vi "vkri801 Assignment_1_XY_Platform.vi"() -> ()   [LabVIEW 2015]
uses:
  <vilib>/DAQmx/create/channels.llb/DAQmx Create Channel (AO-Voltage-Basic).vi
  <vilib>/Utility/error.llb/DialogType.ctl
  <vilib>/DAQmx/create/channels.llb/DAQmx Create Channel (DI-Digital Input).vi
  <vilib>/DAQmx/write.llb/DAQmx Write (Analog DBL 1Chan 1Samp).vi
  <vilib>/DAQmx/read.llb/DAQmx Read (Digital Bool 1Line 1Point).vi
panel:
  in  "Tab Control 2":enum32{"Logistics button"}(tab)
  in  "Motor On/Off":bool
  in  "STOP":bool
  in  "Centre Switch":bool
  in  "Tab Control":enum32{"Pulse Width Graphs"}(tab)
  out "Pulses Left Encoder":dynamicdata(graph) caption="Square"
  out "Pulses Right Encoder":dynamicdata(graph) caption="Square"
  in  "Pulse Width Reset":bool
  in  "Speed Gauges":T1(tab)
  out "Speed Right Motor mm/s":dbl(knob) scale=-50.0..50.0 scale format="%#_6p"
  out "Speed Left Motor mm/s":dbl(knob) scale=-50.0..50.0 scale format="%#_6p"
  out "Y Dimension Speed mm/s 2":dbl(knob) scale=-50.0..50.0 scale format="%#_6p"
  out "X Dimension Speed mm/s 2":dbl(knob) scale=-50.0..50.0 scale format="%#_6p"
  out "LEFT RPM":dbl(knob) scale=-50.0..50.0 scale format="%#_6p"
  out "RIGHT RPM":dbl(knob) scale=-50.0..50.0 scale format="%#_6p"
  in  "Cradle Position":enum32{"Cradle Position"}(tab)
  out "XY Graph 2":cluster{dbl[], dbl[]}(graph)
  in  "Clear Graph":bool
  in  "Chart History":i32=500 caption="Maximum Number of Data Points (Chart History)"
  in  "Read outs":T2(tab)
  out "Left Motor Distance  (mm)":dbl
  out "Right Motor Distance  (mm)":dbl
  out "Right Motor Encoder":dbl
  out "Left Motor Encoder":dbl
  out "Left Motor Frequency":dbl
  out "Right Motor Frequency":dbl
  out "Y":dbl
  out "X":dbl
  out "Y Error":dbl
  out "X Error":dbl
  out "Cursor Y":dbl format="%.2f"
  out "Cursor X":dbl format="%.2f"
  out "X Circle":dbl
  out "Y Circle":dbl
  out "Right Motor Voltage":dbl
  out "Left Motor Voltage":dbl
  in  "Indicator LED":enum32{"Limit Switches"}(tab)
  out "Left":bool
  out "Right":bool
  out "Top":bool
  out "Bottom":bool
  in  "Controls Tab":T3(tab)
  in  "Top Button":bool
  in  "Right Button":bool
  in  "Left Button":bool
  in  "Down Button":bool
  in  "Speed Control":dbl(knob) scale=0.0..10.0
  in  "Left Motor Speed":dbl(knob) scale=-10.0..10.0
  in  "Right Motor Speed":dbl(knob) scale=-10.0..10.0
  in  "Max Voltage":dbl(knob) scale=0.0..10.0
  in  "XY Cursor Graph":cluster{dbl, dbl}[](graph)
  in  "Graph/Coordinate Execute":bool
  in  "K Gain Graph":dbl
  in  "Max Voltage Rectangle":dbl
  in  "Length":dbl
  in  "Width":dbl
  out "Top Left X":dbl
  out "Top Left Y":dbl
  in  "Draw Rectangle":bool
  in  "Y Gain Rectangle":dbl
  in  "X Gain Rectangle":dbl
  in  "Gain Rec":dbl
  in  "Rec Drift Fix":dbl
  in  "Draw Circle":bool
  in  "Reset Circle":bool
  in  "Radius":dbl=-15.0 caption="Amplitude"
  in  "Speed":dbl=0.01 caption="Frequency"
  in  "K Gain Circle":dbl
  in  "X Origin":dbl caption="Offset"
  in  "Y Origin":dbl caption="Offset"
  in  "Channel Selection and Limit Values":T4(tab)
  in  "Right Motor Channel (ao0)":tag="Dev4/ao0"
  in  "Bottom LED":tag="Dev4/ao0"
  in  "Right LED":tag="Dev4/ao0"
  in  "Left LED":tag="Dev4/ao0"
  in  "Left Motor Channel (ao1)":tag="Dev4/ao0"
  in  "Top LED":tag="Dev4/ao0"
  in  "Minimum Voltage":dbl=-6.0
  in  "Maximum Voltage":dbl=6.0
  in  "Rectangle Stop":bool
  in  "Left OK":bool
  in  "Up OK":bool
  in  "Right OK":bool
  in  "Centre Stop":bool
  in  "Numeric Right":dbl
  out "Pulses before refresh\nRight":dbl
  in  "Numeric Left":dbl
  out "Pulses before refresh\nLeft":dbl
  # "Vincent and Mohammad - XY Platform Software"
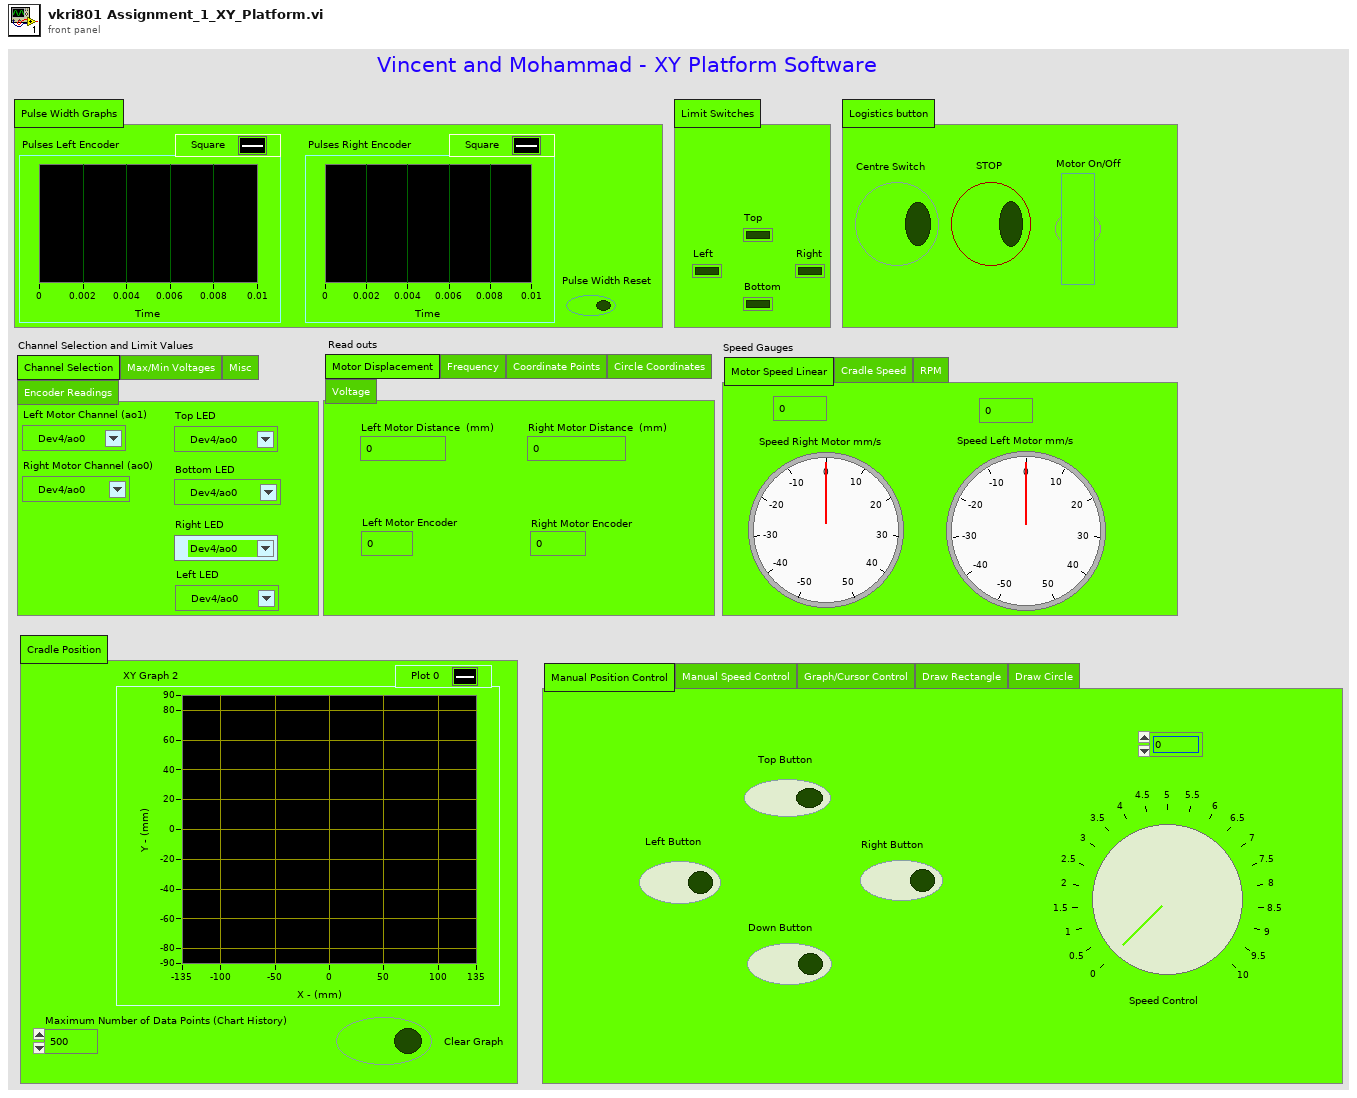
[diagram p1: front panel]
types:
  T1 = enum32{"Motor Speed Linear", "Cradle Speed", "RPM"}
  T2 = enum32{"Motor Displacement", "Frequency", "Coordinate Points", "Circle Coordinates", "Voltage"}
  T3 = enum32{"Manual Position Control", "Manual Speed Control", "Graph/Cursor Control", "Draw Rectangle", "Draw Circle"}
  T4 = enum32{"Channel Selection", "Max/Min Voltages", "Misc", "Encoder Readings"}
  T5 = typedef "DialogType.ctl" = u16
  T6 = typedef "LVPointDoubleTypeDef.ctl" = cluster{"Cursor X":dbl, "Cursor Y":dbl}
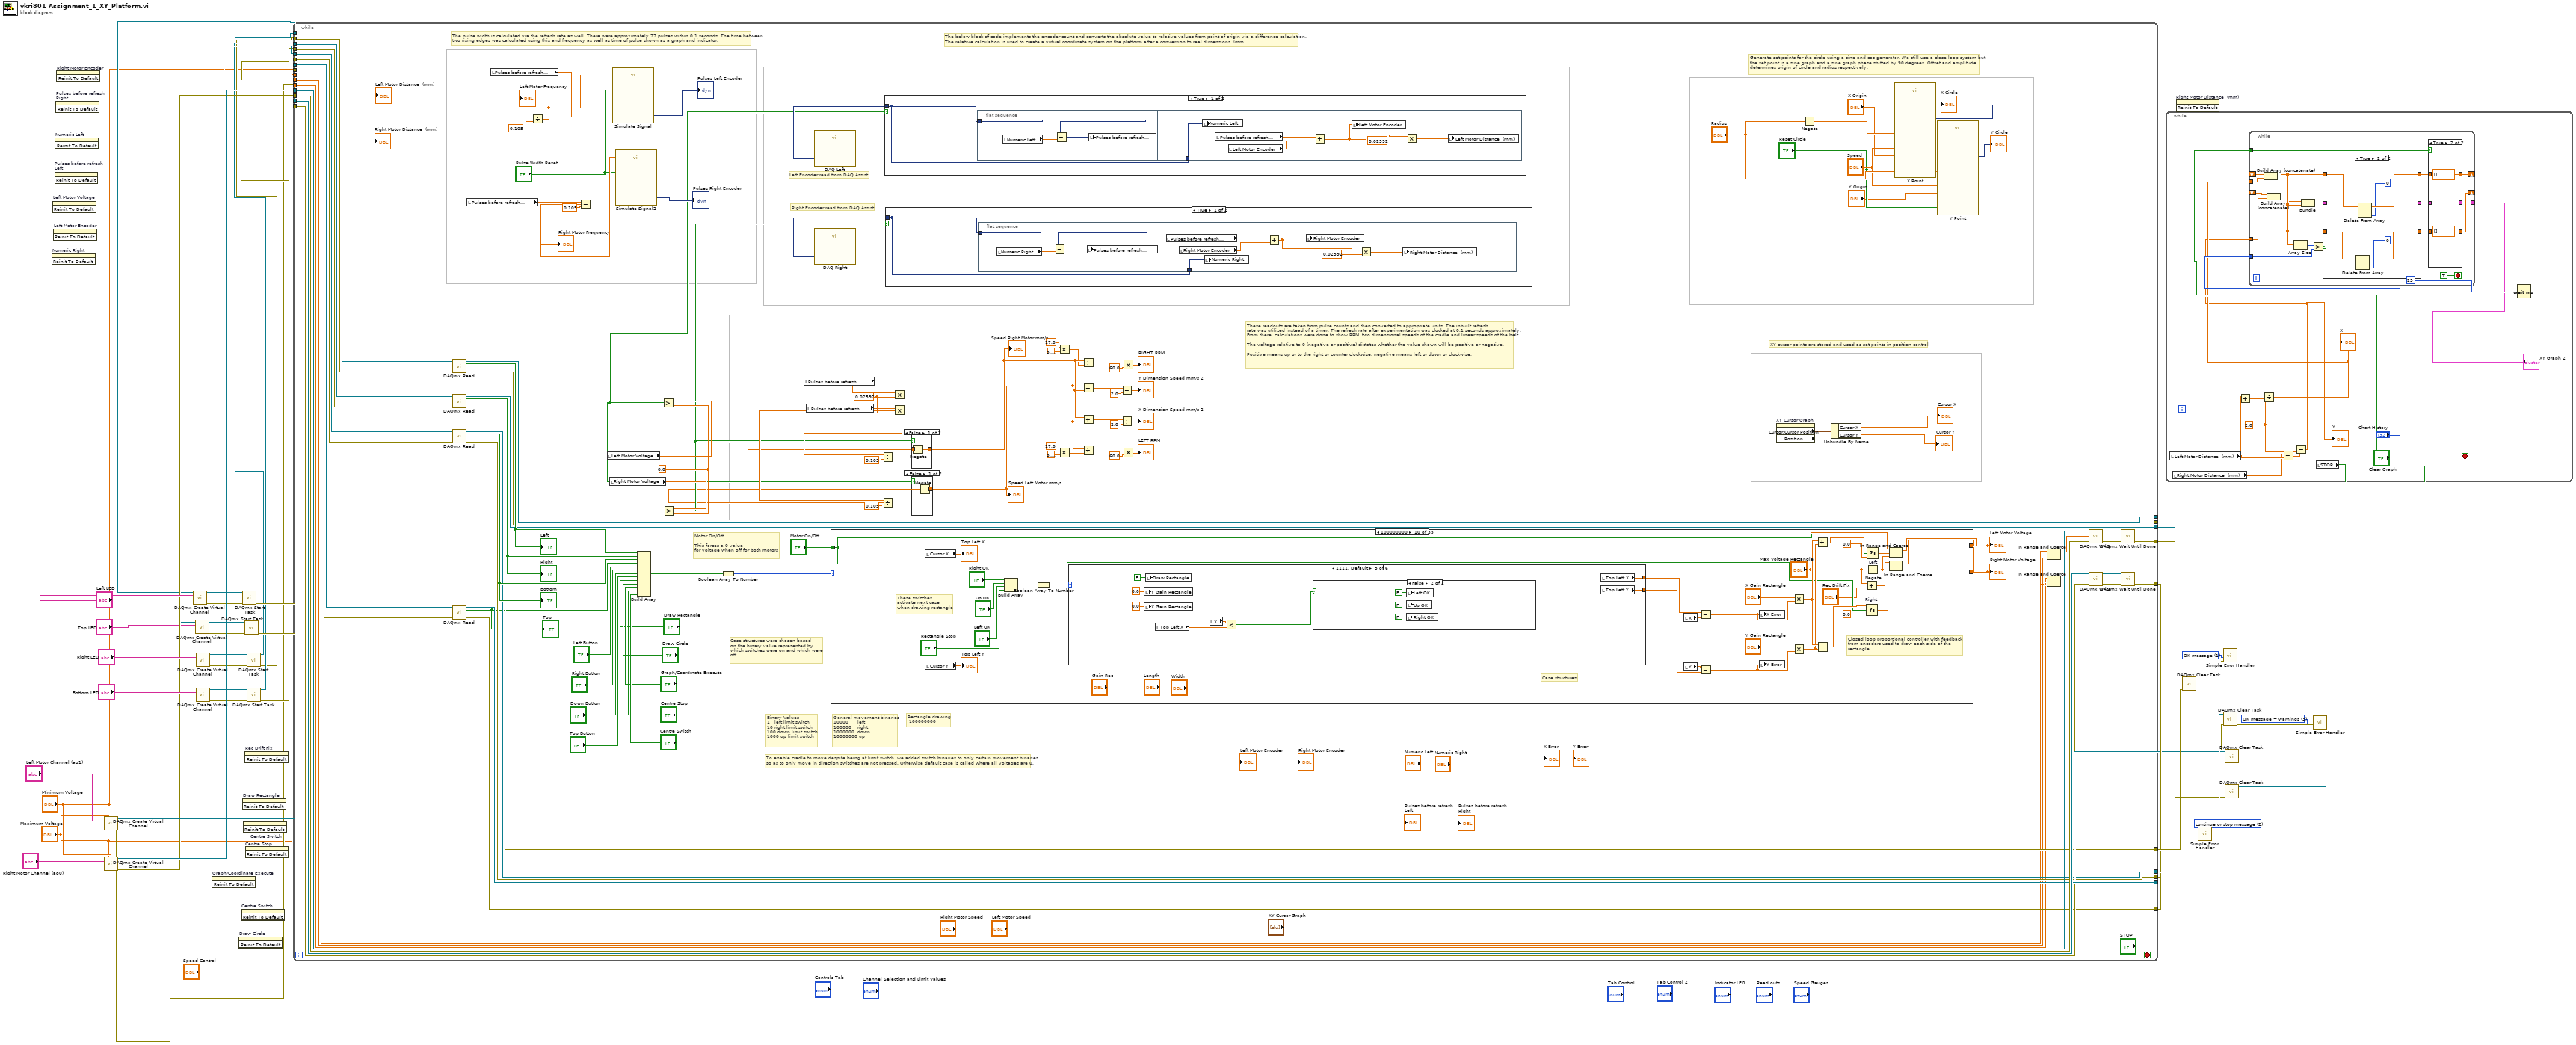
[diagram p0: block diagram]
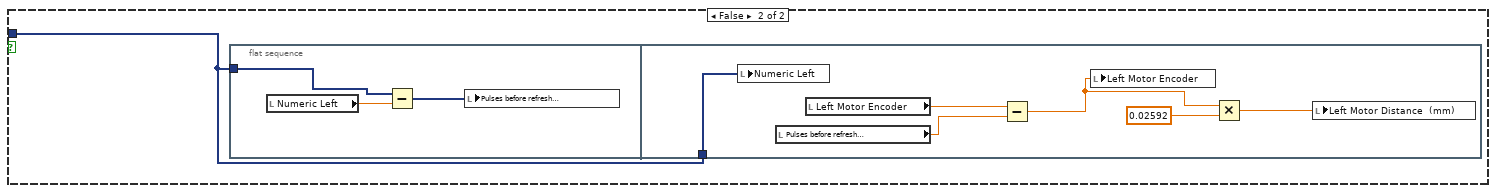
[diagram p6: hidden frame]
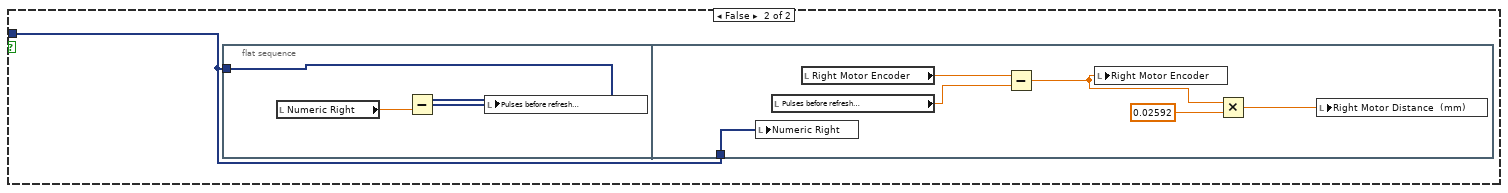
[diagram p7: hidden frame]
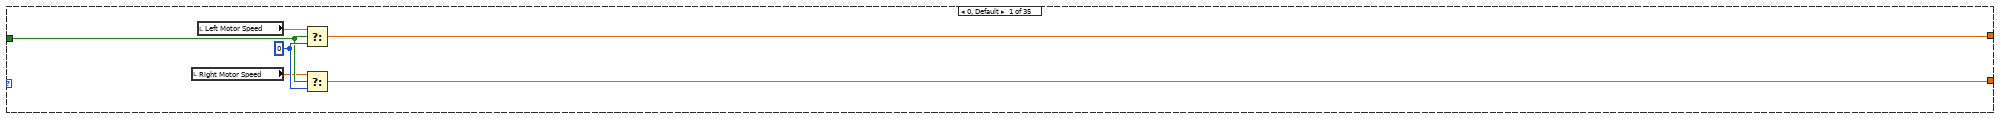
[diagram p8: hidden frame]
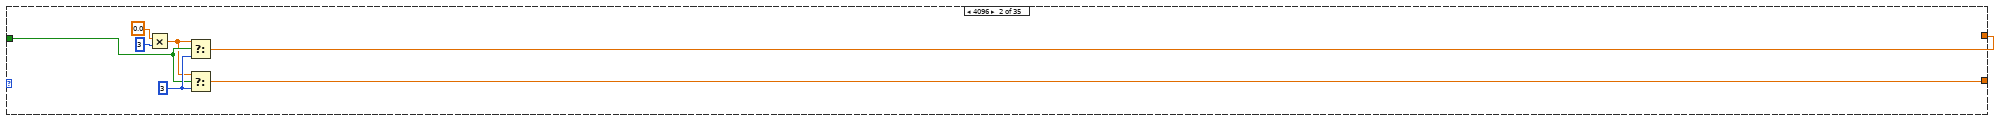
[diagram p9: hidden frame]
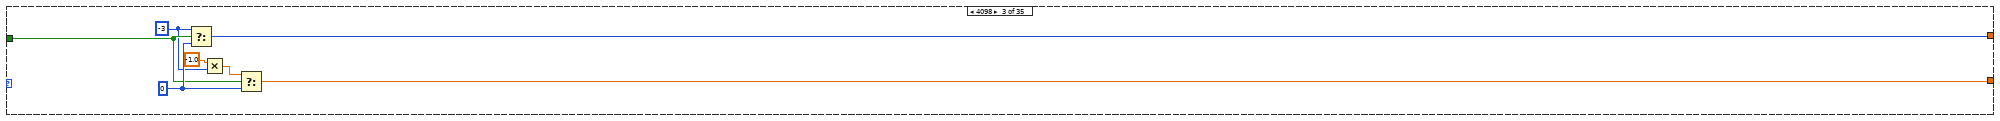
[diagram p10: hidden frame]
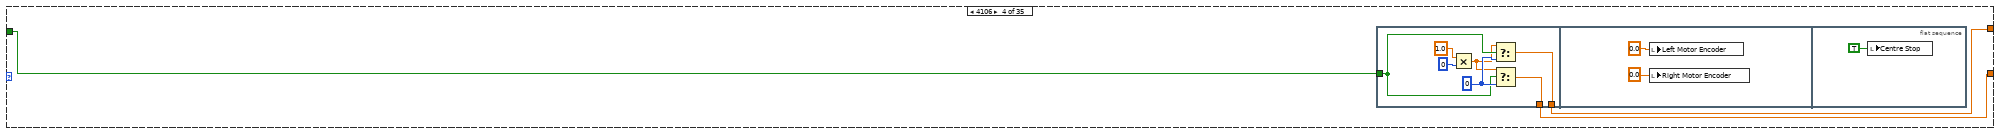
[diagram p11: hidden frame]
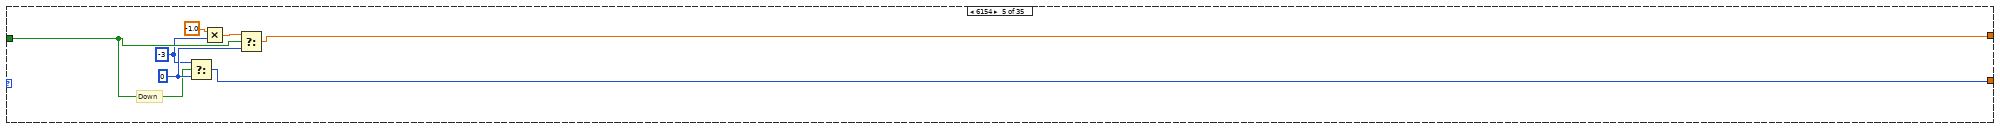
[diagram p12: hidden frame]
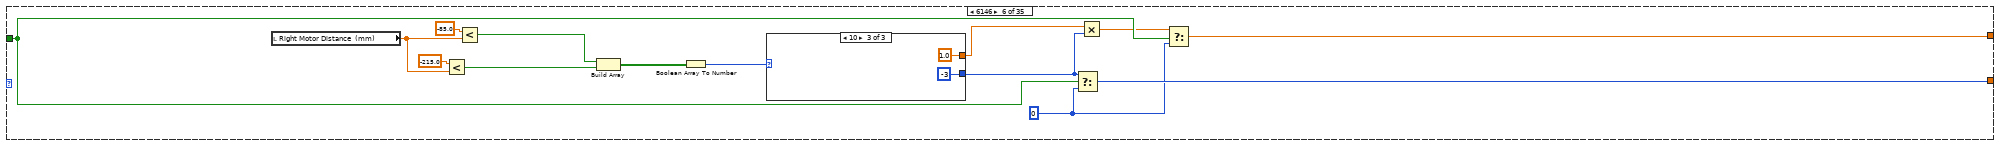
[diagram p13: hidden frame]
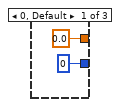
[diagram p14: hidden frame]
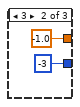
[diagram p15: hidden frame]
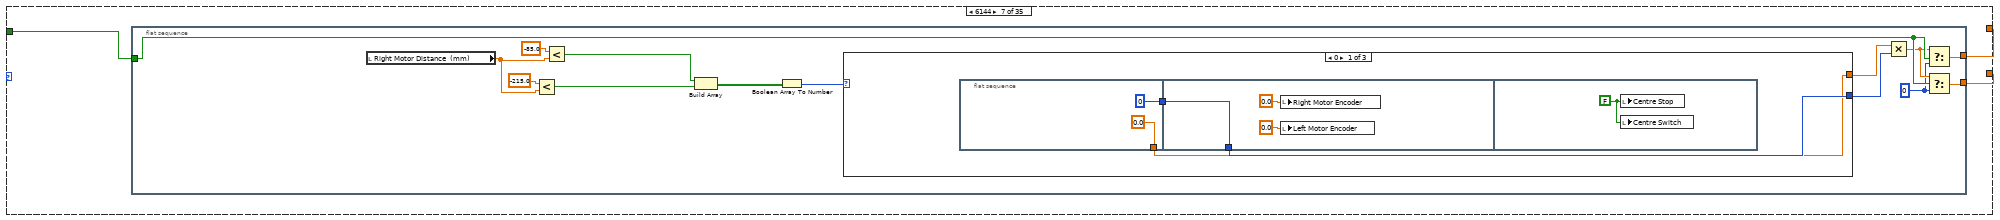
[diagram p16: hidden frame]
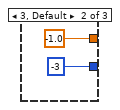
[diagram p17: hidden frame]
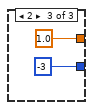
[diagram p18: hidden frame]
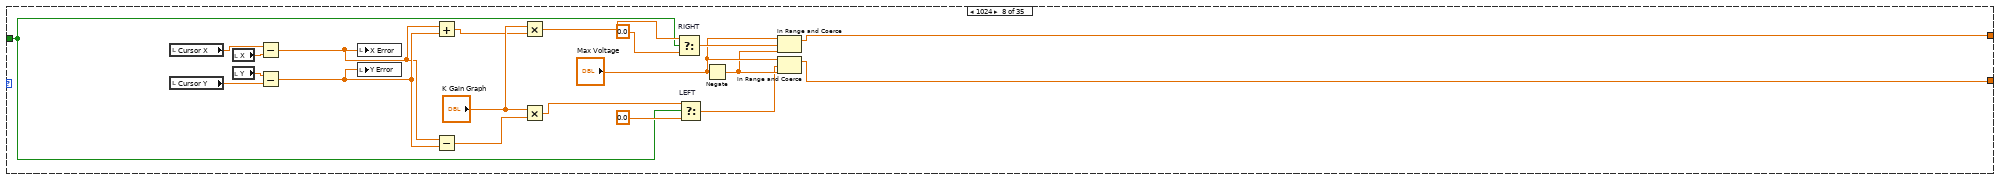
[diagram p19: hidden frame]
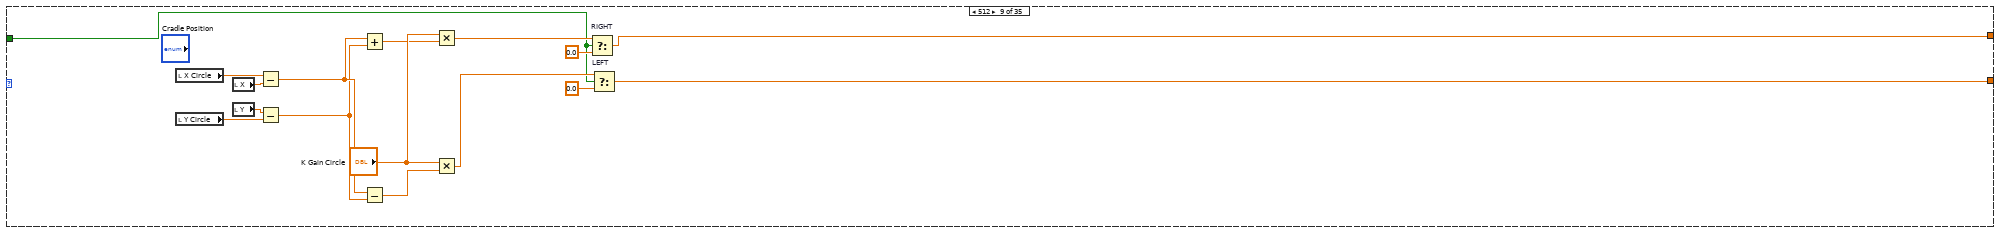
[diagram p20: hidden frame]
diagram:
  w24 = T5 3 items=["no dialog", "OK message", "continue or stop message", "OK message + warnings", "continue/stop + warnings"] ("type of dialog (OK msg:1)")
  w38 = T5 1 items=["no dialog", "OK message", "continue or stop message", "OK message + warnings", "continue/stop + warnings"] ("type of dialog (OK msg:1)")
  w42 = T5 2 items=["no dialog", "OK message", "continue or stop message", "OK message + warnings", "continue/stop + warnings"] ("type of dialog (OK msg:1)")
  n1 = invoke on="Numeric Right" class="DigNum (strict)" method="Reinit To Default"() -> ()  [unwired: 3 in, 3 out]
  n2 = invoke on="Left Motor Voltage" class="DigNum (strict)" method="Reinit To Default"() -> ()  [unwired: 3 in, 3 out]
  n3 = invoke on="Left Motor Encoder" class="DigNum (strict)" method="Reinit To Default"() -> ()  [unwired: 3 in, 3 out]
  n4 = invoke on="Pulses before refresh\nLeft" class="DigNum (strict)" method="Reinit To Default"() -> ()  [unwired: 3 in, 3 out]
  n5 = invoke on="Numeric Left" class="DigNum (strict)" method="Reinit To Default"() -> ()  [unwired: 3 in, 3 out]
  n6 = invoke on="Pulses before refresh\nRight" class="DigNum (strict)" method="Reinit To Default"() -> ()  [unwired: 3 in, 3 out]
  n7 = invoke on="Right Motor Encoder" class="DigNum (strict)" method="Reinit To Default"() -> ()  [unwired: 3 in, 3 out]
  n8 = call-poly <vilib>:"DAQmx Create Virtual Channel.vi"("maximum value"="Maximum Voltage", "minimum value"="Minimum Voltage", "physical channels"="Left Motor Channel (ao1)") -> ("task out"=w37:refnum<k21>, "error out"=w14:errorcluster)  [unwired: 11 in]
  n9 = call-poly <vilib>:"DAQmx Create Virtual Channel.vi"("maximum value"="Maximum Voltage", "minimum value"="Minimum Voltage", "physical channels"="Right Motor Channel (ao0)") -> ("task out"=w40:refnum<k21>, "error out"=w23:errorcluster)  [unwired: 11 in]
  n10 = call-poly <vilib>:"DAQmx Create Virtual Channel.vi"("lines"="Left LED") -> ("task out"=w26:refnum<k21>, "error out"=w27:errorcluster)  [unwired: 13 in]
  n11 = call-poly <vilib>:"DAQmx Create Virtual Channel.vi"("lines"="Top LED") -> ("task out"=w35:refnum<k21>, "error out"=w36:errorcluster)  [unwired: 13 in]
  n12 = call-poly <vilib>:"DAQmx Create Virtual Channel.vi"("lines"="Right LED") -> ("task out"=w29:refnum<k21>, "error out"=w30:errorcluster)  [unwired: 13 in]
  n13 = call-poly <vilib>:"DAQmx Create Virtual Channel.vi"("lines"="Bottom LED") -> ("task out"=w32:refnum<k21>, "error out"=w33:errorcluster)  [unwired: 13 in]
  n14 = invoke on="Graph/Coordinate Execute" class="Bool (strict)" method="Reinit To Default"() -> ()  [unwired: 3 in, 3 out]
  n15 = invoke on="Draw Circle" class="Bool (strict)" method="Reinit To Default"() -> ()  [unwired: 3 in, 3 out]
  n16 = invoke on="Centre Switch" class="Bool (strict)" method="Reinit To Default"() -> ()  [unwired: 3 in, 3 out]
  n17 = call <vilib>:"DAQmx Start Task.vi"("task/channels in"=w26, "error in"=w27) -> ("task out"=w21:refnum<k21>, "error out"=w22:errorcluster)  [unwired: 12 in]
  n18 = invoke on="Draw Rectangle" class="Bool (strict)" method="Reinit To Default"() -> ()  [unwired: 3 in, 3 out]
  n19 = invoke on="Centre Switch" class="Bool (strict)" method="Reinit To Default"() -> ()  [unwired: 3 in, 3 out]
  n20 = call <vilib>:"DAQmx Start Task.vi"("task/channels in"=w35, "error in"=w36) -> ("task out"=w19:refnum<k21>, "error out"=w20:errorcluster)  [unwired: 12 in]
  n21 = invoke on="Rec Drift Fix" class="DigNum (strict)" method="Reinit To Default"() -> ()  [unwired: 3 in, 3 out]
  n22 = invoke on="Centre Stop" class="Bool (strict)" method="Reinit To Default"() -> ()  [unwired: 3 in, 3 out]
  n23 = call <vilib>:"DAQmx Start Task.vi"("task/channels in"=w29, "error in"=w30) -> ("task out"=w15:refnum<k21>, "error out"=w16:errorcluster)  [unwired: 12 in]
  n24 = call <vilib>:"DAQmx Start Task.vi"("task/channels in"=w32, "error in"=w33) -> ("task out"=w17:refnum<k21>, "error out"=w18:errorcluster)  [unwired: 12 in]
  n25 = while {
    tunnel: w40 -> [w148]
    tunnel: w37 -> [w147]
    tunnel: w23 -> [w133]
    tunnel: w22 -> [w132]
    tunnel: w21 -> [w131]
    tunnel: w20 -> [w130]
    tunnel: w19 -> [w129]
    tunnel: w18 -> [w128]
    tunnel: w17 -> [w127]
    tunnel: w16 -> [w126]
    tunnel: w15 -> [w125]
    tunnel: w14 -> [w124]
    tunnel: [w123] -> w13
    tunnel: [w122] -> w12
    tunnel: [w121] -> w11
    tunnel: [w120] -> w10
    tunnel: [w119] -> w9
    tunnel: [w118] -> w8
    tunnel: [w117] -> w7
    tunnel: [w116] -> w6
    tunnel: [w115] -> w5
    tunnel: [w114] -> w4
    tunnel: "Minimum Voltage" -> [w98]
    tunnel: "Maximum Voltage" -> [w97]
    tunnel: "Maximum Voltage" -> [w92]
    stop <- "STOP" stop-if-true
    w82 = 0.02592 ("y")
    w100 = 0.0 ("y")
    # "Rectangle drawing\n 100000000"
    # "To enable cradle to move despite being at limit switch, we added switch binaries to only certain movement binaries\nso as to only move in direction switches are not pressed. Otherwise default case is called where all voltages are 0."
    # "General movement binaries\n10000      left\n100000    right\n1000000  down\n10000000 up"
    # "Binary Values\n1   left limit switch\n10 right limit switch\n100 down limit switch\n1000 up limit switch"
    # "Motor On/Off\n\nThis forces a 0 value\nfor voltage when off for both motors"
    # "Case structures were chosen based \non the binary value represented by\nwhich switches were on and which were\noff."
    # "The pulse width is calculated via the refresh rate as well. There were approximately 77 pulses within 0.1 seconds. The time between \ntwo rising edges was calculated using this and frequency as well as time of pulse shown as a graph and indicator."
    # "These readouts are taken from pulse counts and then converted to appropriate units. The inbuilt refresh\nrate was utilized instead of a timer. The refresh rate after experimentation was clocked at 0.1 seconds approximately.\nFrom there, calculations were done to show RPM, two dimensional speeds of the cradle and linear speeds of the belt.\n\nThe voltage relative to 0 (negative or positive) dictates whether the value shown will be positive or negative. \n\nPositive means up or to the right or counter clockwise, negative means left or down or clockwise."
    # "XY cursor points are stored and used as set points in position control"
    # "Left Encoder read from DAQ Assist"
    # "The below block of code implements the encoder count and converts the absolute value to relative values from point of origin via a difference calculation.\nThe relative calculation is used to create a virtual coordinate system on the platform after a conversion to real dimensions. (mm)"
    # "Generate set points for the circle using a sine and cos generator. We still use a close loop system but \nthe set point is a sine graph and a sine graph phase shifted by 90 degrees. Offset and amplitude \ndetermines origin of circle and radius respectively."
    # "Right Encoder read from DAQ Assist"
    n26 = call-poly <vilib>:"DAQmx Read.vi"("task/channels in"=w131, "error in"=w132) -> ("task out"=w116:refnum<k21>, "data"=w142:bool, "error out"=w115:errorcluster)  [unwired: 11 in]
    "Left" <- w142
    n27 = call-poly <vilib>:"DAQmx Read.vi"("task/channels in"=w125, "error in"=w126) -> ("task out"=w122:refnum<k21>, "data"=w140:bool, "error out"=w121:errorcluster)  [unwired: 11 in]
    "Right" <- w140
    n28 = call-poly <vilib>:"DAQmx Read.vi"("task/channels in"=w127, "error in"=w128) -> ("task out"=w120:refnum<k21>, "data"=w139:bool, "error out"=w119:errorcluster)  [unwired: 11 in]
    "Bottom" <- w139
    n29 = call-poly <vilib>:"DAQmx Read.vi"("task/channels in"=w129, "error in"=w130) -> ("task out"=w118:refnum<k21>, "data"=w113:bool, "error out"=w117:errorcluster)  [unwired: 11 in]
    "Top" <- w113
    n30 = local read "Pulses before refresh\nRight"() -> (w71:dbl)
    n31 = local read "Pulses before refresh\nLeft"() -> (w75:dbl)
    n32 = Divide(x=w75, y=0.105) -> (x/y=w73:dbl)
    "Left Motor Frequency" <- w73
    n33 = Divide(x=w71, y=0.105) -> (x/y=w70:dbl)
    "Right Motor Frequency" <- w70
    n34 = local read "Left Motor Voltage"() -> (w103:dbl)
    n35 = local read "Right Motor Voltage"() -> (w101:dbl)
    n36 = call "Simulate Signal"("Reset Signal"="Pulse Width Reset", "Frequency"=w73) -> ("Square"=→"Pulses Left Encoder":dynamicdata)  [unwired: 12 in, 1 out]
    n37 = call "Simulate Signal2"("Reset Signal"="Pulse Width Reset", "Frequency"=w70) -> ("Square"=→"Pulses Right Encoder":dynamicdata)  [unwired: 12 in, 1 out]
    n38 = Build Array(w142, w140, w139, w113, "Left Button", "Right Button", "Down Button", "Top Button", "Draw Rectangle", "Draw Circle", "Graph/Coordinate Execute", "Centre Stop", "Centre Switch") -> (w141:bool[])
    n39 = Greater?(x=w103, y=w100) -> (0:w65:bool)
    n40 = Greater?(x=w101, y=w100) -> (0:w66:bool)
    n41 = Boolean Array To Number(Boolean array=w141) -> (number=w111:u32)
    n42 = local read "Pulses before refresh\nRight"() -> (w80:dbl)
    n43 = local read "Pulses before refresh\nLeft"() -> (w81:dbl)
    n44 = call "DAQ Left"() -> ("data"=w104:dynamicdata)  [unwired: 16 in, 3 out]
    n45 = call "DAQ Right"() -> ("data"=w102:dynamicdata)  [unwired: 16 in, 3 out]
    n46 = case shown="100000000" w111 {
      tunnel: [w200 w207 w214 w217 w234 w248 w257 w290 w307 w340 w430 w437 w444 w451 w458 w465 w472 w479 w486 w493 w500 w507 w514 w521 w528 w535 w542 w549 w556 w563 w570 w576 w582 w588 w594] -> w94
      tunnel: [w199 w206 w213 w216 w233 w247 w256 w291 w308 w342 w429 w436 w443 w450 w457 w464 w471 w478 w485 w492 w499 w506 w513 w520 w527 w534 w541 w548 w555 w562 w569 w575 w581 w587 w593] -> w96
      tunnel: "Motor On/Off" -> [w197 w204 w211 w215 w231 w246 w255 w298 w314 w330 w427 w434 w441 w448 w455 w462 w469 w476 w483 w490 w497 w504 w511 w518 w525 w532 w539 w546 w553 w560 w567 w573 w579 w585 w591]
      frame 0, Default {
        w198 = 0
        n47 = local read "Right Motor Speed"() -> (w196:dbl)
        n48 = local read "Left Motor Speed"() -> (w195:dbl)
        n49 = Select(t=w195, s=w197, f=w198) -> (s? t:f=w199:dbl)
        n50 = Select(t=w196, s=w197, f=w198) -> (s? t:f=w200:dbl)
      }
      frame 4096 {
        w205 = 3
        n51 = Multiply(x=0.0, y=3) -> (x*y=w202:dbl)
        n52 = Select(t=w202, s=w204, f=w205) -> (s? t:f=w206:dbl)
        n53 = Select(t=w202, s=w204, f=w205) -> (s? t:f=w207:dbl)
      }
      frame 4098 {
        w208 = -3
        w212 = 0
        n54 = Select(t=w208, s=w211, f=w212) -> (s? t:f=w213:i32)
        n55 = Multiply(x=-1.0, y=w208) -> (x*y=w209:dbl)
        n56 = Select(t=w209, s=w211, f=w212) -> (s? t:f=w214:dbl)
      }
      frame 4106 {
        n57 = flat-sequence {
          tunnel: [w224] -> w217
          tunnel: [w223] -> w216
          tunnel: w215 -> [w221]
          frame #0 {
            w222 = 0
            n58 = Multiply(x=1.0, y=0) -> (x*y=w219:dbl)
            n59 = Select(t=w219, s=w221, f=w222) -> (s? t:f=w223:dbl)
            n60 = Select(t=w219, s=w221, f=w222) -> (s? t:f=w224:dbl)
          }
          frame #1 {
            n61 = local write "Left Motor Encoder"(0.0 ("Left Motor Encoder")) -> ()
            n62 = local write "Right Motor Encoder"(0.0 ("Right Motor Encoder")) -> ()
          }
          frame #2 {
            n63 = local write "Centre Stop"(TRUE) -> ()
          }
        }
      }
      frame 6154 {
        w228 = -3
        w232 = 0
        # "Down"
        n64 = Select(t=w228, s=w231, f=w232) -> (s? t:f=w234:i32)
        n65 = Multiply(x=-1.0, y=w228) -> (x*y=w229:dbl)
        n66 = Select(t=w229, s=w231, f=w232) -> (s? t:f=w233:dbl)
      }
      frame 6146 {
        w238 = 0
        n67 = local read "Right Motor Distance  (mm)"() -> (w235:dbl)
        n68 = Less?(x=-215.0, y=w235) -> (x < y?=w240:bool)
        n69 = Less?(x=-85.0, y=w235) -> (x < y?=w242:bool)
        n70 = Build Array(w242, w240) -> (w244:bool[])
        n71 = Boolean Array To Number(Boolean array=w244) -> (number=w243:u32)
        n72 = case shown="10" w243 {
          tunnel: [0 -3 -3] -> w237
          tunnel: [0.0 ("x") -1.0 ("x") 1.0 ("x")] -> w236
          frame 0, Default {
          }
          frame 3 {
          }
          frame 2 {
          }
        }
        n73 = Select(t=w237, s=w246, f=w238) -> (s? t:f=w248:i32)
        n74 = Multiply(x=w236, y=w237) -> (x*y=w245:dbl)
        n75 = Select(t=w245, s=w246, f=w238) -> (s? t:f=w247:dbl)
      }
      frame 6144 {
        n76 = flat-sequence {
          tunnel: [w271] -> w257
          tunnel: [w270] -> w256
          tunnel: w255 -> [w269]
          frame #0 {
            w259 = 0
            n77 = local read "Right Motor Distance  (mm)"() -> (w260:dbl)
            n78 = Less?(x=-215.0, y=w260) -> (x < y?=w262:bool)
            n79 = Less?(x=-85.0, y=w260) -> (x < y?=w264:bool)
            n80 = Build Array(w264, w262) -> (w266:bool[])
            n81 = Boolean Array To Number(Boolean array=w266) -> (number=w265:u32)
            n82 = case shown="0" w265 {
              tunnel: [w273 -3 -3] -> w267
              tunnel: [w272 -1.0 ("x") 1.0 ("x")] -> w258
              frame 0 {
                n83 = flat-sequence {
                  tunnel: [0] -> w274
                  tunnel: [0.0 ("x")] -> w272
                  tunnel: w274 -> [w277]
                  tunnel: [w277] -> w273
                  frame #0 {
                  }
                  frame #1 {
                    n84 = local write "Right Motor Encoder"(0.0 ("Right Motor Encoder")) -> ()
                    n85 = local write "Left Motor Encoder"(0.0 ("Left Motor Encoder")) -> ()
                  }
                  frame #2 {
                    w280 = FALSE
                    n86 = local write "Centre Stop"(w280) -> ()
                    n87 = local write "Centre Switch"(w280) -> ()
                  }
                }
              }
              frame 3, Default {
              }
              frame 2 {
              }
            }
            n88 = Multiply(x=w258, y=w267) -> (x*y=w268:dbl)
            n89 = Select(t=w268, s=w269, f=w259) -> (s? t:f=w270:dbl)
            n90 = Select(t=w268, s=w269, f=w259) -> (s? t:f=w271:dbl)
          }
        }
      }
      frame 1024 {
        n91 = local read "Cursor X"() -> (w295:dbl)
        n92 = local read "Cursor Y"() -> (w296:dbl)
        n93 = local read "X"() -> (w294:dbl)
        n94 = local read "Y"() -> (w297:dbl)
        n95 = Subtract(x=w295, y=w294) -> (x-y=w285:dbl)
        n96 = Subtract(x=w297, y=w296) -> (x-y=w286:dbl)
        n97 = local write "X Error"(w285) -> ()
        n98 = local write "Y Error"(w286) -> ()
        n99 = Add(x=w285, y=w286) -> (x+y=w293:dbl)
        n100 = Subtract(x=w285, y=w286) -> (x-y=w304:dbl)
        n101 = Multiply(x="K Gain Graph", y=w293) -> (x*y=w302:dbl)
        n102 = Multiply(x="K Gain Graph", y=w304) -> (x*y=w301:dbl)
        n103 = Select "RIGHT"(t=w302, s=w298, f=0.0) -> (s? t:f=w292:dbl)
        n104 = Select "LEFT"(t=w301, s=w298, f=0.0) -> (s? t:f=w287:dbl)
        n105 = Negate(x="Max Voltage") -> (-x=w288:dbl)
        n106 = In Range and Coerce(upper limit="Max Voltage", x=w292, lower limit=w288) -> (coerced(x)=w291:dbl)  [unwired: 1 out]
        n107 = In Range and Coerce(upper limit="Max Voltage", x=w287, lower limit=w288) -> (coerced(x)=w290:dbl)  [unwired: 1 out]
      }
      frame 512 {
        n108 = local read "X Circle"() -> (w306:dbl)
        n109 = local read "Y Circle"() -> (w305:dbl)
        n110 = local read "X"() -> (w312:dbl)
        n111 = local read "Y"() -> (w313:dbl)
        n112 = Subtract(x=w306, y=w312) -> (x-y=w310:dbl)
        n113 = Subtract(x=w313, y=w305) -> (x-y=w309:dbl)
        n114 = Add(x=w310, y=w309) -> (x+y=w311:dbl)
        n115 = Subtract(x=w310, y=w309) -> (x-y=w320:dbl)
        n116 = Multiply(x="K Gain Circle", y=w311) -> (x*y=w318:dbl)
        n117 = Multiply(x="K Gain Circle", y=w320) -> (x*y=w317:dbl)
        n118 = Select "RIGHT"(t=w318, s=w314, f=0.0) -> (s? t:f=w308:dbl)
        n119 = Select "LEFT"(t=w317, s=w314, f=0.0) -> (s? t:f=w307:dbl)
      }
      frame 256 {
        # "Case structures"
        # "Closed loop proportional controller with feedback\nfrom encoders used to draw each side of the \nrectangle."
        # "These switches\nactivate next case\nwhen drawing rectangle"
        n120 = local read "Cursor X"() -> (→"Top Left X":dbl)
        n121 = local read "Cursor Y"() -> (→"Top Left Y":dbl)
        n122 = Build Array("Right OK", "Up OK", "Left OK", "Rectangle Stop") -> (w347:bool[])
        n123 = Boolean Array To Number(Boolean array=w347) -> (number=w346:u32)
        n124 = case shown="1111, Default" w346 {
          tunnel: [w362 w366 w380 w390 w399 w413] -> w345
          tunnel: [w359 w374 w378 w391 w400 w414] -> w344
          frame 0 {
            n125 = local write "X Gain Rectangle"(0.0 ("X Gain Rectangle")) -> ()
            n126 = local read "Top Left Y"() -> (w356:dbl)
            n127 = local read "Gain Rec"() -> (w357:dbl)
            n128 = local write "Y Gain Rectangle"(w357) -> ()
            n129 = local read "Width"() -> (w355:dbl)
            n130 = Subtract(x=w356, y=w355) -> (x-y=w354:dbl)
            n131 = local read "Y"() -> (w353:dbl)
            n132 = Less?(x=w353, y=w354) -> (x < y?=w352:bool)
            n133 = case shown="False" w352 {
              frame False {
              }
              frame True {
                n134 = local write "Right OK"(TRUE ("Right OK")) -> ()
              }
            }
            n135 = local read "Top Left Y"() -> (w360:dbl)
            n136 = local read "Width"() -> (w361:dbl)
            n137 = local read "Top Left X"() -> (w362:dbl)
            n138 = Subtract(x=w360, y=w361) -> (x-y=w359:dbl)
          }
          frame 1 {
            n139 = local write "Y Gain Rectangle"(0.0 ("Y Gain Rectangle")) -> ()
            n140 = local read "Top Left X"() -> (w373:dbl)
            n141 = local read "Gain Rec"() -> (w365:dbl)
            n142 = local read "Length"() -> (w372:dbl)
            n143 = local write "X Gain Rectangle"(w365) -> ()
            n144 = Add(x=w373, y=w372) -> (x+y=w371:dbl)
            n145 = local read "X"() -> (w370:dbl)
            n146 = Greater?(x=w370, y=w371) -> (0:w369:bool)
            n147 = case shown="False" w369 {
              frame False {
              }
              frame True {
                n148 = local write "Up OK"(TRUE ("Right OK")) -> ()
              }
            }
            n149 = local read "Top Left Y"() -> (w375:dbl)
            n150 = local read "Top Left X"() -> (w368:dbl)
            n151 = local read "Length"() -> (w367:dbl)
            n152 = local read "Width"() -> (w376:dbl)
            n153 = Add(x=w368, y=w367) -> (x+y=w366:dbl)
            n154 = Subtract(x=w375, y=w376) -> (x-y=w374:dbl)
          }
          frame 3 {
            n155 = local write "X Gain Rectangle"(0.0 ("X Gain Rectangle")) -> ()
            n156 = local read "Top Left Y"() -> (w379:dbl)
            n157 = local read "Gain Rec"() -> (w385:dbl)
            n158 = local write "Y Gain Rectangle"(w385) -> ()
            n159 = local read "Y"() -> (w384:dbl)
            n160 = Greater?(x=w384, y=w379) -> (0:w383:bool)
            n161 = case shown="False" w383 {
              frame False {
              }
              frame True {
                n162 = local write "Left OK"(TRUE ("Right OK")) -> ()
              }
            }
            n163 = local read "Top Left X"() -> (w382:dbl)
            n164 = local read "Length"() -> (w381:dbl)
            n165 = local read "Top Left Y"() -> (w378:dbl)
            n166 = Add(x=w382, y=w381) -> (x+y=w380:dbl)
          }
          frame 7 {
            n167 = local write "Y Gain Rectangle"(0.0 ("Y Gain Rectangle")) -> ()
            n168 = local read "Top Left X"() -> (w392:dbl)
            n169 = local read "Gain Rec"() -> (w388:dbl)
            n170 = local write "X Gain Rectangle"(w388) -> ()
            n171 = local read "X"() -> (w394:dbl)
            n172 = Less?(x=w394, y=w392) -> (x < y?=w393:bool)
            n173 = case shown="True" w393 {
              frame False {
              }
              frame True {
                n174 = local write "Rectangle Stop"(TRUE ("Right OK")) -> ()
              }
            }
            n175 = local read "Top Left X"() -> (w390:dbl)
            n176 = local read "Top Left Y"() -> (w391:dbl)
          }
          frame 15, Default {
            n177 = local write "Y Gain Rectangle"(0.0 ("Y Gain Rectangle")) -> ()
            n178 = local write "X Gain Rectangle"(0.0 ("X Gain Rectangle")) -> ()
            n179 = local write "Draw Rectangle"(FALSE ("Draw Rectangle")) -> ()
            n180 = local read "Top Left X"() -> (w401:dbl)
            n181 = local read "X"() -> (w403:dbl)
            n182 = Less?(x=w403, y=w401) -> (x < y?=w402:bool)
            n183 = case shown="False" w402 {
              frame True {
                n184 = local write "Left OK"(FALSE ("Right OK")) -> ()
                n185 = local write "Up OK"(FALSE ("Up OK")) -> ()
                n186 = local write "Right OK"(FALSE ("Right OK")) -> ()
              }
              frame False {
                n187 = local write "Left OK"(FALSE ("Right OK")) -> ()
                n188 = local write "Up OK"(FALSE ("Up OK")) -> ()
                n189 = local write "Right OK"(FALSE ("Right OK")) -> ()
              }
            }
            n190 = local read "Top Left X"() -> (w399:dbl)
            n191 = local read "Top Left Y"() -> (w400:dbl)
          }
          frame 8 {
            n192 = local write "Y Gain Rectangle"(0.0 ("Y Gain Rectangle")) -> ()
            n193 = local write "X Gain Rectangle"(0.0 ("X Gain Rectangle")) -> ()
            n194 = local write "Rectangle Stop"(FALSE ("OK Button 2")) -> ()
            n195 = local read "Top Left X"() -> (w415:dbl)
            n196 = local read "X"() -> (w417:dbl)
            n197 = Less?(x=w417, y=w415) -> (x < y?=w416:bool)
            n198 = case shown="True" w416 {
              frame True {
                n199 = local write "Left OK"(FALSE ("Right OK")) -> ()
                n200 = local write "Up OK"(FALSE ("Up OK")) -> ()
                n201 = local write "Right OK"(FALSE ("Right OK")) -> ()
              }
              frame False {
                n202 = local write "Left OK"(FALSE ("Right OK")) -> ()
                n203 = local write "Up OK"(FALSE ("Up OK")) -> ()
                n204 = local write "Right OK"(FALSE ("Right OK")) -> ()
              }
            }
            n205 = local read "Top Left X"() -> (w413:dbl)
            n206 = local read "Top Left Y"() -> (w414:dbl)
          }
        }
        n207 = local read "X"() -> (w348:dbl)
        n208 = local read "Y"() -> (w349:dbl)
        n209 = Subtract(x=w345, y=w348) -> (x-y=w331:dbl)
        n210 = Subtract(x=w349, y=w344) -> (x-y=w332:dbl)
        n211 = local write "X Error"(w331) -> ()
        n212 = local write "Y Error"(w332) -> ()
        n213 = Multiply(x="X Gain Rectangle", y=w331) -> (x*y=w334:dbl)
        n214 = Multiply(x="Y Gain Rectangle", y=w332) -> (x*y=w333:dbl)
        n215 = Add(x=w334, y=w333) -> (x+y=w337:dbl)
        n216 = Subtract(x=w334, y=w333) -> (x-y=w338:dbl)
        n217 = Add(x="Max Voltage Rectangle", y="Rec Drift Fix") -> (x+y=w328:dbl)
        n218 = Select "Right"(t=w338, s=w330, f=0.0) -> (s? t:f=w341:dbl)
        n219 = Select "Left"(t=w337, s=w330, f=0.0) -> (s? t:f=w343:dbl)
        n220 = Negate(x="Max Voltage Rectangle") -> (-x=w339:dbl)
        n221 = In Range and Coerce(upper limit="Max Voltage Rectangle", x=w343, lower limit=w339) -> (coerced(x)=w342:dbl)  [unwired: 1 out]
        n222 = In Range and Coerce(upper limit=w328, x=w341, lower limit=w339) -> (coerced(x)=w340:dbl)  [unwired: 1 out]
      }
      frame 128 {
        w428 = 0
        n223 = local read "Speed Control"() -> (w426:dbl)
        n224 = Select(t=w426, s=w427, f=w428) -> (s? t:f=w430:dbl)
        n225 = Multiply(x=-1.0, y=w426) -> (x*y=w424:dbl)
        n226 = Select(t=w424, s=w427, f=w428) -> (s? t:f=w429:dbl)
      }
      frame 129 {
        w435 = 0
        n227 = local read "Speed Control"() -> (w433:dbl)
        n228 = Select(t=w433, s=w434, f=w435) -> (s? t:f=w437:dbl)
        n229 = Multiply(x=-1.0, y=w433) -> (x*y=w431:dbl)
        n230 = Select(t=w431, s=w434, f=w435) -> (s? t:f=w436:dbl)
      }
      frame 130 {
        w442 = 0
        n231 = local read "Speed Control"() -> (w440:dbl)
        n232 = Select(t=w440, s=w441, f=w442) -> (s? t:f=w444:dbl)
        n233 = Multiply(x=-1.0, y=w440) -> (x*y=w438:dbl)
        n234 = Select(t=w438, s=w441, f=w442) -> (s? t:f=w443:dbl)
      }
      frame 132 {
        w449 = 0
        n235 = local read "Speed Control"() -> (w447:dbl)
        n236 = Select(t=w447, s=w448, f=w449) -> (s? t:f=w451:dbl)
        n237 = Multiply(x=-1.0, y=w447) -> (x*y=w445:dbl)
        n238 = Select(t=w445, s=w448, f=w449) -> (s? t:f=w450:dbl)
      }
      frame 133 {
        w456 = 0
        n239 = local read "Speed Control"() -> (w454:dbl)
        n240 = Select(t=w454, s=w455, f=w456) -> (s? t:f=w458:dbl)
        n241 = Multiply(x=-1.0, y=w454) -> (x*y=w452:dbl)
        n242 = Select(t=w452, s=w455, f=w456) -> (s? t:f=w457:dbl)
      }
      frame 64 {
        w463 = 0
        n243 = local read "Speed Control"() -> (w460:dbl)
        n244 = Select(t=w460, s=w462, f=w463) -> (s? t:f=w464:dbl)
        n245 = Multiply(x=-1.0, y=w460) -> (x*y=w459:dbl)
        n246 = Select(t=w459, s=w462, f=w463) -> (s? t:f=w465:dbl)
      }
      frame 74 {
        w470 = 0
        n247 = local read "Speed Control"() -> (w467:dbl)
        n248 = Select(t=w467, s=w469, f=w470) -> (s? t:f=w471:dbl)
        n249 = Multiply(x=-1.0, y=w467) -> (x*y=w466:dbl)
        n250 = Select(t=w466, s=w469, f=w470) -> (s? t:f=w472:dbl)
      }
      frame 65 {
        w477 = 0
        n251 = local read "Speed Control"() -> (w474:dbl)
        n252 = Select(t=w474, s=w476, f=w477) -> (s? t:f=w478:dbl)
        n253 = Multiply(x=-1.0, y=w474) -> (x*y=w473:dbl)
        n254 = Select(t=w473, s=w476, f=w477) -> (s? t:f=w479:dbl)
      }
      frame 66 {
        w484 = 0
        n255 = local read "Speed Control"() -> (w481:dbl)
        n256 = Select(t=w481, s=w483, f=w484) -> (s? t:f=w485:dbl)
        n257 = Multiply(x=-1.0, y=w481) -> (x*y=w480:dbl)
        n258 = Select(t=w480, s=w483, f=w484) -> (s? t:f=w486:dbl)
      }
      frame 72 {
        w491 = 0
        n259 = local read "Speed Control"() -> (w488:dbl)
        n260 = Select(t=w488, s=w490, f=w491) -> (s? t:f=w492:dbl)
        n261 = Multiply(x=-1.0, y=w488) -> (x*y=w487:dbl)
        n262 = Select(t=w487, s=w490, f=w491) -> (s? t:f=w493:dbl)
      }
      frame 32 {
        w498 = 0
        n263 = local read "Speed Control"() -> (w495:dbl)
        n264 = Multiply(x=1.0, y=w495) -> (x*y=w494:dbl)
        n265 = Select(t=w494, s=w497, f=w498) -> (s? t:f=w499:dbl)
        n266 = Select(t=w494, s=w497, f=w498) -> (s? t:f=w500:dbl)
      }
      frame 33 {
        w505 = 0
        n267 = local read "Speed Control"() -> (w502:dbl)
        n268 = Multiply(x=1.0, y=w502) -> (x*y=w501:dbl)
        n269 = Select(t=w501, s=w504, f=w505) -> (s? t:f=w506:dbl)
        n270 = Select(t=w501, s=w504, f=w505) -> (s? t:f=w507:dbl)
      }
      frame 36 {
        w512 = 0
        n271 = local read "Speed Control"() -> (w509:dbl)
        n272 = Multiply(x=1.0, y=w509) -> (x*y=w508:dbl)
        n273 = Select(t=w508, s=w511, f=w512) -> (s? t:f=w513:dbl)
        n274 = Select(t=w508, s=w511, f=w512) -> (s? t:f=w514:dbl)
      }
      frame 40 {
        w519 = 0
        n275 = local read "Speed Control"() -> (w516:dbl)
        n276 = Multiply(x=1.0, y=w516) -> (x*y=w515:dbl)
        n277 = Select(t=w515, s=w518, f=w519) -> (s? t:f=w520:dbl)
        n278 = Select(t=w515, s=w518, f=w519) -> (s? t:f=w521:dbl)
      }
      frame 37 {
        w526 = 0
        n279 = local read "Speed Control"() -> (w523:dbl)
        n280 = Multiply(x=1.0, y=w523) -> (x*y=w522:dbl)
        n281 = Select(t=w522, s=w525, f=w526) -> (s? t:f=w527:dbl)
        n282 = Select(t=w522, s=w525, f=w526) -> (s? t:f=w528:dbl)
      }
      frame 16 {
        w533 = 0
        n283 = local read "Speed Control"() -> (w530:dbl)
        n284 = Multiply(x=-1.0, y=w530) -> (x*y=w529:dbl)
        n285 = Select(t=w529, s=w532, f=w533) -> (s? t:f=w534:dbl)
        n286 = Select(t=w529, s=w532, f=w533) -> (s? t:f=w535:dbl)
      }
      frame 18 {
        w540 = 0
        n287 = local read "Speed Control"() -> (w537:dbl)
        n288 = Multiply(x=-1.0, y=w537) -> (x*y=w536:dbl)
        n289 = Select(t=w536, s=w539, f=w540) -> (s? t:f=w541:dbl)
        n290 = Select(t=w536, s=w539, f=w540) -> (s? t:f=w542:dbl)
      }
      frame 20 {
        w547 = 0
        n291 = local read "Speed Control"() -> (w544:dbl)
        n292 = Multiply(x=-1.0, y=w544) -> (x*y=w543:dbl)
        n293 = Select(t=w543, s=w546, f=w547) -> (s? t:f=w548:dbl)
        n294 = Select(t=w543, s=w546, f=w547) -> (s? t:f=w549:dbl)
      }
      frame 24 {
        w554 = 0
        n295 = local read "Speed Control"() -> (w551:dbl)
        n296 = Multiply(x=-1.0, y=w551) -> (x*y=w550:dbl)
        n297 = Select(t=w550, s=w553, f=w554) -> (s? t:f=w555:dbl)
        n298 = Select(t=w550, s=w553, f=w554) -> (s? t:f=w556:dbl)
      }
      frame 17 {
        w561 = 0
        n299 = local read "Speed Control"() -> (w558:dbl)
        n300 = Multiply(x=0.0, y=w558) -> (x*y=w557:dbl)
        n301 = Select(t=w557, s=w560, f=w561) -> (s? t:f=w562:dbl)
        n302 = Select(t=w557, s=w560, f=w561) -> (s? t:f=w563:dbl)
      }
      frame 26 {
        w568 = 0
        n303 = local read "Speed Control"() -> (w565:dbl)
        n304 = Multiply(x=0.0, y=w565) -> (x*y=w564:dbl)
        n305 = Select(t=w564, s=w567, f=w568) -> (s? t:f=w569:dbl)
        n306 = Select(t=w564, s=w567, f=w568) -> (s? t:f=w570:dbl)
      }
      frame 8 {
        w574 = 0
        # "When up switch is pressed, voltages go to zero."
        n307 = Select(t=0, s=w573, f=w574) -> (s? t:f=w575:i32)
        n308 = Select(t=0, s=w573, f=w574) -> (s? t:f=w576:i32)
      }
      frame 4 {
        w580 = 0
        # "When down switch is pressed, voltages go to zero."
        n309 = Select(t=0, s=w579, f=w580) -> (s? t:f=w581:i32)
        n310 = Select(t=0, s=w579, f=w580) -> (s? t:f=w582:i32)
      }
      frame 2 {
        w586 = 0
        # "When right switch is pressed, voltages go to zero."
        n311 = Select(t=0, s=w585, f=w586) -> (s? t:f=w587:i32)
        n312 = Select(t=0, s=w585, f=w586) -> (s? t:f=w588:i32)
      }
      frame 1 {
        w592 = 0
        # "When left limit switch is hit and no other buttons pressed, voltage is forced to zero."
        n313 = Select(t=0, s=w591, f=w592) -> (s? t:f=w593:i32)
        n314 = Select(t=0, s=w591, f=w592) -> (s? t:f=w594:i32)
      }
    }
    "Left Motor Voltage" <- w96
    "Right Motor Voltage" <- w94
    n315 = case shown="True" w65 {
      tunnel: w104 -> [w155 w165]
      frame True {
        n316 = flat-sequence {
          tunnel: w155 -> [w158]
          tunnel: w155 -> [w164]
          frame #0 {
            n317 = local read "Numeric Left"() -> (w157:dbl)
            n318 = Subtract(x=w158, y=w157) -> (x-y=w156:dynamicdata)
            n319 = local write "Pulses before refresh\nLeft"(w156) -> ()
          }
          frame #1 {
            n320 = local write "Numeric Left"(w164) -> ()
            n321 = local read "Pulses before refresh\nLeft"() -> (w163:dbl)
            n322 = local read "Left Motor Encoder"() -> (w162:dbl)
            n323 = Add(x=w163, y=w162) -> (x+y=w160:dbl)
            n324 = local write "Left Motor Encoder"(w160) -> ()
            n325 = Multiply(x=w160, y=0.02592) -> (x*y=w159:dbl)
            n326 = local write "Left Motor Distance  (mm)"(w159) -> ()
          }
        }
      }
      frame False {
        n327 = flat-sequence {
          tunnel: w165 -> [w168]
          tunnel: w165 -> [w174]
          frame #0 {
            n328 = local read "Numeric Left"() -> (w167:dbl)
            n329 = Subtract(x=w168, y=w167) -> (x-y=w166:dynamicdata)
            n330 = local write "Pulses before refresh\nLeft"(w166) -> ()
          }
          frame #1 {
            n331 = local write "Numeric Left"(w174) -> ()
            n332 = local read "Pulses before refresh\nLeft"() -> (w173:dbl)
            n333 = local read "Left Motor Encoder"() -> (w172:dbl)
            n334 = Subtract(x=w172, y=w173) -> (x-y=w170:dbl)
            n335 = local write "Left Motor Encoder"(w170) -> ()
            n336 = Multiply(x=w170, y=0.02592) -> (x*y=w169:dbl)
            n337 = local write "Left Motor Distance  (mm)"(w169) -> ()
          }
        }
      }
    }
    n338 = case shown="True" w66 {
      tunnel: w102 -> [w175 w185]
      frame True {
        n339 = flat-sequence {
          tunnel: w175 -> [w178]
          tunnel: w175 -> [w184]
          frame #0 {
            n340 = local read "Numeric Right"() -> (w177:dbl)
            n341 = Subtract(x=w178, y=w177) -> (x-y=w176:dynamicdata)
            n342 = local write "Pulses before refresh\nRight"(w176) -> ()
          }
          frame #1 {
            n343 = local read "Pulses before refresh\nRight"() -> (w183:dbl)
            n344 = local read "Right Motor Encoder"() -> (w182:dbl)
            n345 = local write "Numeric Right"(w184) -> ()
            n346 = Add(x=w183, y=w182) -> (x+y=w180:dbl)
            n347 = local write "Right Motor Encoder"(w180) -> ()
            n348 = Multiply(x=w180, y=0.02592) -> (x*y=w179:dbl)
            n349 = local write "Right Motor Distance  (mm)"(w179) -> ()
          }
        }
      }
      frame False {
        n350 = flat-sequence {
          tunnel: w185 -> [w188]
          tunnel: w185 -> [w194]
          frame #0 {
            n351 = local read "Numeric Right"() -> (w187:dbl)
            n352 = Subtract(x=w188, y=w187) -> (x-y=w186:dynamicdata)
            n353 = local write "Pulses before refresh\nRight"(w186) -> ()
          }
          frame #1 {
            n354 = local write "Numeric Right"(w194) -> ()
            n355 = local read "Pulses before refresh\nRight"() -> (w193:dbl)
            n356 = local read "Right Motor Encoder"() -> (w192:dbl)
            n357 = Subtract(x=w192, y=w193) -> (x-y=w190:dbl)
            n358 = local write "Right Motor Encoder"(w190) -> ()
            n359 = Multiply(x=w190, y=0.02592) -> (x*y=w189:dbl)
            n360 = local write "Right Motor Distance  (mm)"(w189) -> ()
          }
        }
      }
    }
    n361 = Multiply(x=w80, y=w82) -> (x*y=w78:dbl)
    n362 = Divide(x=w78, y=0.105) -> (x/y=w64:dbl)
    n363 = Multiply(x=w81, y=w82) -> (x*y=w77:dbl)
    n364 = Divide(x=w77, y=0.105) -> (x/y=w63:dbl)
    n365 = case shown="False" w66 {
      tunnel: w64 -> [w153 w154]
      tunnel: [w152 w154] -> w56
      frame False {
        n366 = Negate(x=w153) -> (-x=w152:dbl)
      }
      frame True {
      }
    }
    "Speed Right Motor mm/s" <- w56
    n367 = case shown="False" w65 {
      tunnel: w63 -> [w150 w151]
      tunnel: [w149 w151] -> w45
      frame False {
        n368 = Negate(x=w150) -> (-x=w149:dbl)
      }
      frame True {
      }
    }
    "Speed Left Motor mm/s" <- w45
    n369 = Multiply(x=17.0, y=3.141592653589793) -> (x*y=w55:dbl)
    n370 = Multiply(x=17.0, y=3.141592653589793) -> (x*y=w50:dbl)
    n371 = Divide(x=w56, y=w55) -> (x/y=w53:dbl)
    n372 = Subtract(x=w45, y=w56) -> (x-y=w58:dbl)
    n373 = Add(x=w56, y=w45) -> (x+y=w61:dbl)
    n374 = Divide(x=w45, y=w50) -> (x/y=w48:dbl)
    n375 = Divide(x=w58, y=2.0) -> (x/y=→"Y Dimension Speed mm/s 2":dbl)
    n376 = Divide(x=w61, y=2.0) -> (x/y=→"X Dimension Speed mm/s 2":dbl)
    n377 = Multiply(x=w53, y=60.0) -> (x*y=→"RIGHT RPM":dbl)
    n378 = Multiply(x=w48, y=60.0) -> (x*y=→"LEFT RPM":dbl)
    n379 = property on="XY Cursor Graph" class="XYGraph (strict)" props=["Cursor", "Cursor Position", "Position"]() -> ("Cursor.Cursor Position"=w110:T6)  [unwired: 2 in, 3 out]
    n380 = Negate(x="Radius") -> (-x=w89:dbl)
    n381 = Unbundle By Name(w110) -> ("Cursor X"=→"Cursor X":dbl, "Cursor Y"=→"Cursor Y":dbl)
    n382 = call "X Point"("Offset"="X Origin", "Reset Signal"="Reset Circle", "Frequency"="Speed", "Amplitude"=w89) -> ("Sine"=→"X Circle":dynamicdata)  [unwired: 10 in, 1 out]
    n383 = call "Y Point"("Offset"="Y Origin", "Reset Signal"="Reset Circle", "Frequency"="Speed", "Amplitude"="Radius") -> ("Sine"=→"Y Circle":dynamicdata)  [unwired: 10 in, 1 out]
    n384 = In Range and Coerce(upper limit=w97, x=w96, lower limit=w98) -> (coerced(x)=w95:dbl)  [unwired: 1 out]
    n385 = In Range and Coerce(upper limit=w92, x=w94, lower limit=w98) -> (coerced(x)=w93:dbl)  [unwired: 1 out]
    n386 = call-poly <vilib>:"DAQmx Write.vi"("task/channels in"=w147, "data"=w95, "error in"=w124) -> ("task out"=w144:refnum<k21>, "error out"=w143:errorcluster)  [unwired: 10 in, 1 out]
    n387 = call-poly <vilib>:"DAQmx Write.vi"("task/channels in"=w148, "data"=w93, "error in"=w133) -> ("task out"=w146:refnum<k21>, "error out"=w145:errorcluster)  [unwired: 10 in, 1 out]
    n388 = call <vilib>:"DAQmx Wait Until Done.vi"("task/channels in"=w144, "error in"=w143) -> ("error out"=w123:errorcluster)  [unwired: 12 in, 1 out]
    n389 = call <vilib>:"DAQmx Wait Until Done.vi"("task/channels in"=w146, "error in"=w145) -> ("error out"=w114:errorcluster)  [unwired: 12 in, 1 out]
  }
  n390 = while {
    stop <- w600 stop-if-true
    w603 = 2.0 ("y")
    n391 = local read "Left Motor Distance  (mm)"() -> (w602:dbl)
    n392 = local read "Right Motor Distance  (mm)"() -> (w601:dbl)
    n393 = Add(x=w602, y=w601) -> (x+y=w605:dbl)
    n394 = Divide(x=w605, y=w603) -> (x/y=w596:dbl)
    "X" <- w596
    n395 = Subtract(x=w601, y=w602) -> (x-y=w604:dbl)
    n396 = Divide(x=w604, y=w603) -> (x/y=w595:dbl)
    "Y" <- w595
    n397 = while {
      tunnel: w596 -> [w624]
      tunnel: w595 -> [w622]
      shift-right: [w611] -> _
      shift-left: _ -> [w623]
      shift-right: [w614] -> _
      shift-left: _ -> [w621]
      tunnel: "Chart History" -> [w619]
      tunnel: [w609] -> w599
      tunnel: "Clear Graph" -> [w607]
      stop <- TRUE stop-if-true
      n398 = Build Array (concatenate)(w623, w624) -> (w613:dbl[])
      n399 = Build Array (concatenate)(w621, w622) -> (w616:dbl[])
      n400 = Array Size(array=w616) -> (size(s)=w620:i32)
      n401 = Bundle(w613, w616) -> (w617:cluster{dbl[], dbl[]})  [unwired: 1 in]
      n402 = Greater?(x=w620, y=w619) -> (0:w618:bool)
      n403 = case shown="True" w618 {
        tunnel: w617 -> [w631 w634]
        tunnel: w616 -> [w633 w636]
        tunnel: [w633 w635] -> w615
        tunnel: [w632 w639] -> w612
        tunnel: w613 -> [w632 w640]
        tunnel: [w631 w634] -> w610
        frame False {
        }
        frame True {
          n404 = Delete From Array(array=w636, index=0) -> (array with subset deleted=w635:dbl[])  [unwired: 1 in, 1 out]
          n405 = Delete From Array(array=w640, index=0) -> (array with subset deleted=w639:dbl[])  [unwired: 1 in, 1 out]
        }
      }
      n406 = case shown="True" w607 {
        tunnel: w615 -> [w627 _]
        tunnel: [w627 dbl[] []] -> w614
        tunnel: w612 -> [w626 _]
        tunnel: [w626 dbl[] []] -> w611
        tunnel: [w625 w628] -> w609
        tunnel: w610 -> [w625 w628]
        frame False {
        }
        frame True {
        }
      }
    }
    "XY Graph 2" <- w599
    n407 = local read "STOP"() -> (w600:bool)
    n408 = Wait (ms)(milliseconds to wait=u32 25) -> ()  [unwired: 1 out]
  }
  n409 = invoke on="Right Motor Distance  (mm)" class="DigNum (strict)" method="Reinit To Default"() -> ()  [unwired: 3 in, 3 out]
  n410 = call <vilib>:"DAQmx Clear Task.vi"("task in"=w12, "error in"=w11) -> ()  [unwired: 13 in, 1 out]
  n411 = call <vilib>:"Simple Error Handler.vi"("type of dialog (OK msg:1)"=w42, "error in (no error)"=w4) -> ()  [unwired: 3 in, 5 out]
  n412 = call <vilib>:"Simple Error Handler.vi"("type of dialog (OK msg:1)"=w38, "error in (no error)"=w13) -> ()  [unwired: 3 in, 5 out]
  n413 = call <vilib>:"DAQmx Clear Task.vi"("task in"=w10, "error in"=w9) -> ("error out"=w25:errorcluster)  [unwired: 13 in]
  n414 = call <vilib>:"DAQmx Clear Task.vi"("task in"=w8, "error in"=w7) -> ()  [unwired: 13 in, 1 out]
  n415 = call <vilib>:"DAQmx Clear Task.vi"("task in"=w6, "error in"=w5) -> ()  [unwired: 13 in, 1 out]
  n416 = call <vilib>:"Simple Error Handler.vi"("type of dialog (OK msg:1)"=w24, "error in (no error)"=w25) -> ()  [unwired: 3 in, 5 out]
